vi "Global_Stop_Scan.vi"() -> ()   [LabVIEW 2018]
panel:
  in  "Stop Scan":bool
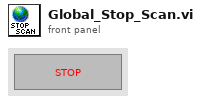
[diagram p1: front panel]
diagram:
